vi "write_fifo_resonance_FF_FB.vi"(5 "enable fly-back reversion?":bool, 6 "invert channels":bool[](array[boolean])=[FALSE, FALSE], 7 "fly-back?":bool, 8 "pixel finished?":bool, 10 "maximum bit depth":i8, 11 "integration cluster in":T1) -> (0 "FIFO overflow out":bool, 3 "integration cluster out":T1)   [LabVIEW 2010]
uses:
  integration_cluster.ctl
  <vilib>/rvi/DataTransferAndStorage/Container/XNode/niFpgaContainer.xnode
  <vilib>/rvi/DataTransferAndStorage/Container/Common/niFpgaContainerMethod.ctl
  <vilib>/rvi/DataTransferAndStorage/Container/Common/niFpgaTransferTypeControl.ctl
  <vilib>/rvi/Memory/Memory_Emulation/nirvimemoryEmulationManagerCache_GetValue.vi
  <vilib>/rvi/DataTransferAndStorage/Container/Common/niFpgaContainerGetUniqueNameForEmu.vi
  <vilib>/rvi/Memory/Memory_Emulation/nirvimemoryEmulationManagerCache_InsertValue.vi
  <vilib>/Utility/error.llb/Clear Errors.vi
  <vilib>/rvi/Memory/Memory_Emulation/nirvimemoryEmulationManagerCache_SetValue.vi
  <vilib>/rvi/interface/RandomDataEmulation/nirviRandomDataFPGAFIFO.vi
  <vilib>/rvi/interface/RandomDataEmulation/niFpgaRandomDataHandleErrors.vi
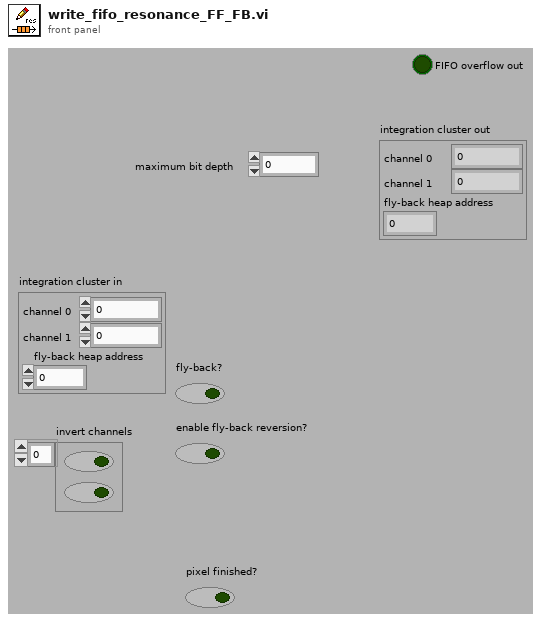
[diagram p1: front panel]
types:
  T1 = typedef "integration_cluster.ctl" = cluster{"channel 0":u32, "channel 1":u32, "fly-back heap address":u32}
  T2 = typedef "niFpgaContainerMethod.ctl" = enum16{"<none>", "write", "read", "clear", "getNumberOfElementsToWrite", "getNumberOfElementsToRead", "enable", "disable", "flushAndDisable", "getStreamState", "readA", "readB", "dramWrite", "dramWriteWithByteEnables", "dramRequestData", "dramRetrieveData"}
  T3 = typedef "niFpgaTransferTypeControl.ctl" = enum16{"Target-Scoped", "Host to Target - DMA", "Target to Host - DMA", "Peer to Peer Reader", "Peer to Peer Writer", "Bidirectional"}
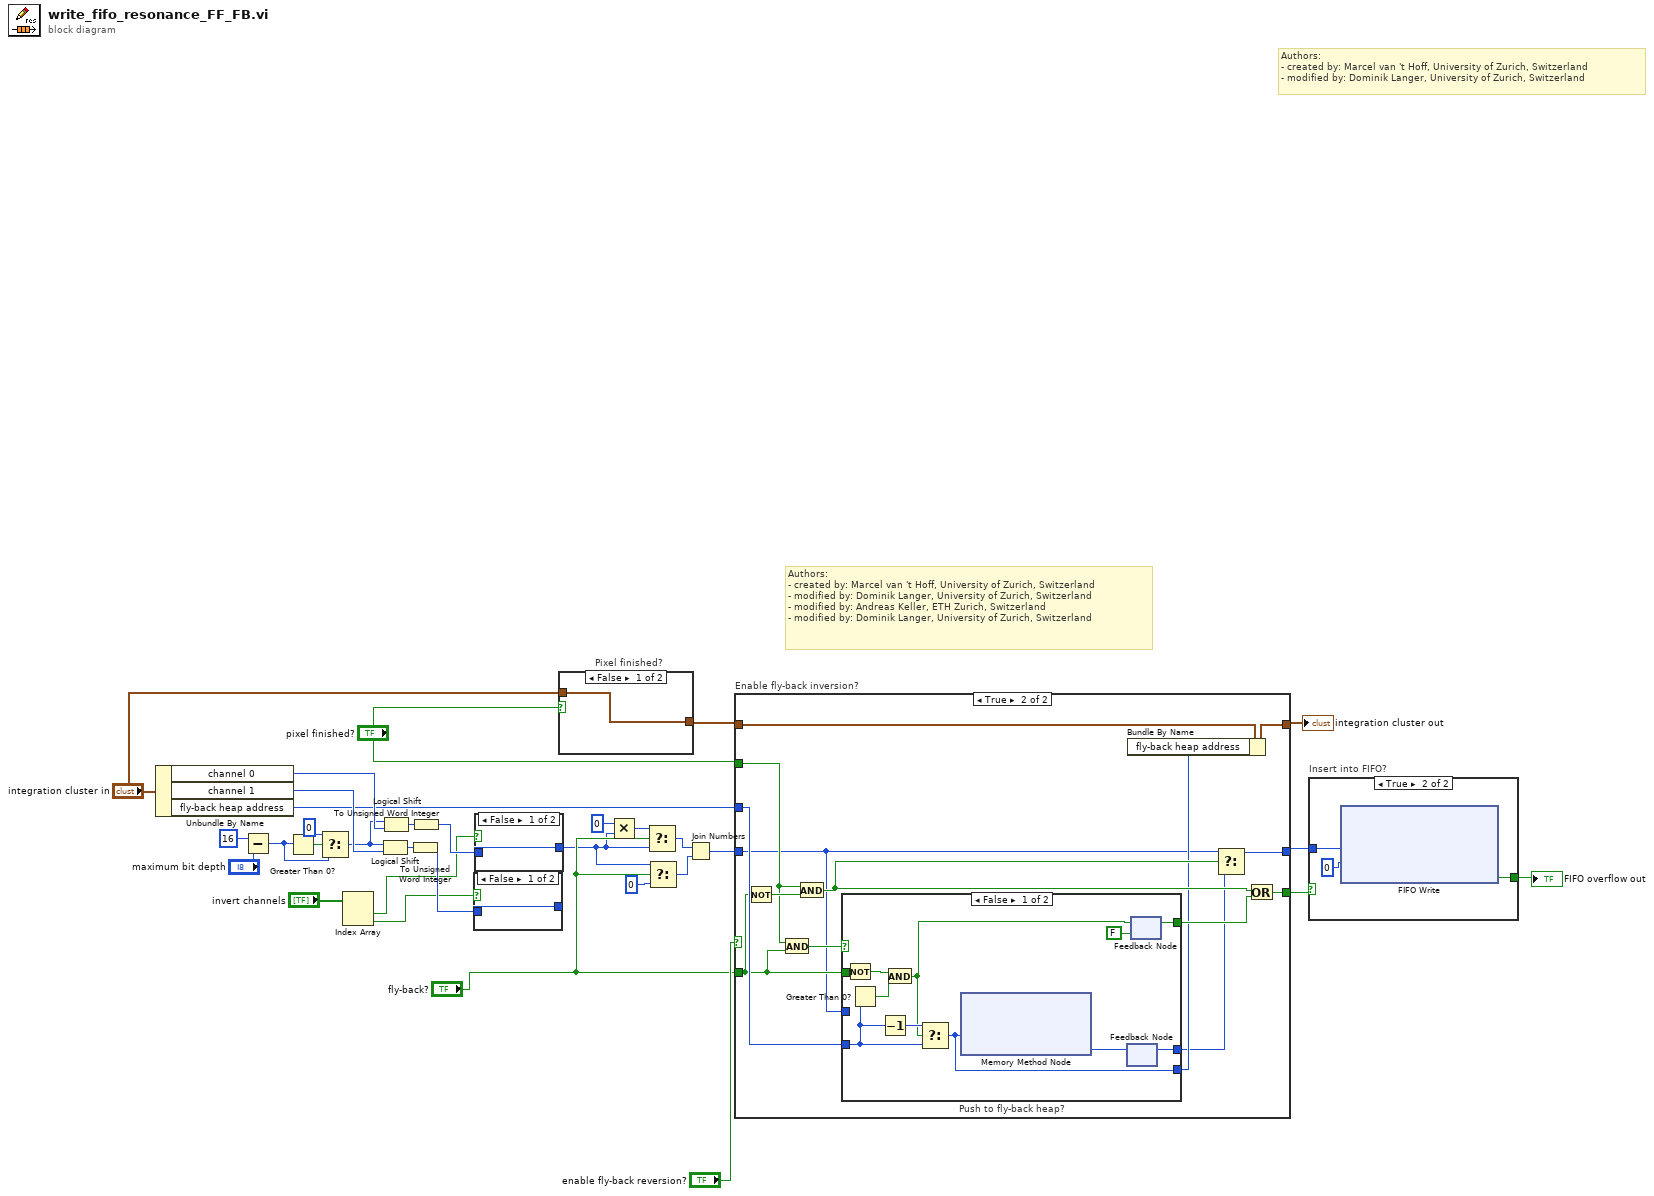
[diagram p0: block diagram]
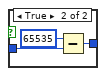
[diagram p2: hidden frame]
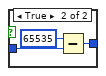
[diagram p3: hidden frame]
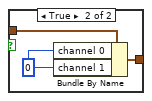
[diagram p4: hidden frame]
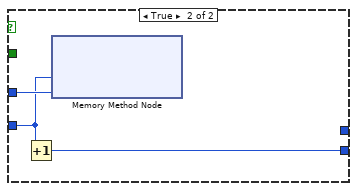
[diagram p6: hidden frame]
diagram:
  # "Authors: \n- created by: Marcel van 't Hoff, University of Zurich, Switzerland\n- modified by: Dominik Langer, University of Zurich, Switzerland\n- modified by: Andreas Keller, ETH Zurich, Switzerland\n- modified by: Dominik Langer, University of Zurich, Switzerland"
  # "Authors: \n- created by: Marcel van 't Hoff, University of Zurich, Switzerland\n- modified by: Dominik Langer, University of Zurich, Switzerland"
  n1 = Unbundle By Name("integration cluster in") -> ("channel 0"=w25:u32, "channel 1"=w26:u32, "fly-back heap address"=w19:u32)
  n2 = Subtract(x=i8 16, y="maximum bit depth") -> (x-y=w28:i8)
  n3 = Greater Than 0?(x=w28) -> (x > 0?=w27:bool)
  n4 = Select(t=i8 0 ("f"), s=w27, f=w28) -> (s? t:f=w24:i8)
  n5 = Index Array(array="invert channels") -> (element #1=w10:bool, element #2=w9:bool)  [unwired: 2 in]
  n6 = Logical Shift(y=w24, x=w26) -> (x << y=w23:u32)
  n7 = Logical Shift(y=w24, x=w25) -> (x << y=w22:u32)
  n8 = To Unsigned Word Integer(number=w23) -> (unsigned 16bit integer=w12:u16)
  n9 = To Unsigned Word Integer(number=w22) -> (unsigned 16bit integer=w13:u16)
  n10 = case shown="False" w9 {
    tunnel: [w33 w35] -> _
    tunnel: w12 -> [w33 w34]
    frame False {
    }
    frame True {
      n11 = Subtract(x=u16 65535, y=w34) -> (x-y=w35:u16)
    }
  }
  n12 = case shown="False" w10 {
    tunnel: [w37 w39] -> w3
    tunnel: w13 -> [w37 w38]
    frame False {
    }
    frame True {
      n13 = Subtract(x=u16 65535, y=w38) -> (x-y=w39:u16)
    }
  }
  n14 = case "Pixel finished?" shown="False" "pixel finished?" {
    tunnel: "integration cluster in" -> [w41 w43]
    tunnel: [w41 w42] -> w16
    frame False {
    }
    frame True {
      w44 = u32 0 ("channel 1")
      n15 = Bundle By Name(cluster=w43, "channel 0"=w44, "channel 1"=w44) -> (w42:T1)
    }
  }
  n16 = Multiply(x=u16 0, y=w3) -> (x*y=w7:u16)
  n17 = Select(t=w7, s="fly-back?", f=w3) -> (s? t:f=w8:u16)
  n18 = Select(t=w3, s="fly-back?", f=u16 0 ("x")) -> (s? t:f=w4:u16)
  n19 = Join Numbers(hi=w8, lo=w4) -> ((hi.lo)=w1:u32)
  n20 = case "Enable fly-back inversion?" shown="True" "enable fly-back reversion?" {
    tunnel: w19 -> [_ w61]
    tunnel: w1 -> [w47 w50]
    tunnel: [w47 w59] -> w21
    tunnel: "pixel finished?" -> [w46 w54]
    tunnel: [w46 w49] -> w18
    tunnel: "fly-back?" -> [_ w56]
    tunnel: w16 -> [w45 w53]
    tunnel: [w45 w51] -> w14
    frame False {
    }
    frame True {
      n21 = Not(x=w56) -> (.not. x?=w60:bool)
      n22 = And(x=w54, y=w56) -> (x .and. y?=w58:bool)
      n23 = And(x=w54, y=w60) -> (x .and. y?=w57:bool)
      n24 = case "Push to fly-back heap?" shown="False" w58 {
        tunnel: w50 -> [_ w201]
        tunnel: [w64 w200] -> w52
        tunnel: w61 -> [w66 w199]
        tunnel: w56 -> [w71 _]
        tunnel: [w68 _] -> w48
        tunnel: [w70 _] -> w55
        frame False {
          n25 = Not(x=w71) -> (.not. x?=w63:bool)
          n26 = Greater Than 0?(x=w66) -> (x > 0?=w72:bool)
          n27 = Decrement(x=w66) -> (x-1=w65:u32)
          n28 = And(x=w63, y=w72) -> (x .and. y?=w62:bool)
          n29 = Select(t=w65, s=w62, f=w66) -> (s? t:f=w64:u32)
          n30 = xnode ("Memory Method Node")("Address"=w64) -> ("Data"=w67:u32)  [unwired: 1 in, 1 out]
          n31 = feedback #1() -> (w68:u32)  [unwired: 1 in]
          n32 = feedback-in #1(w67) -> ()
          n33 = feedback #2(FALSE) -> (w70:bool)
          n34 = feedback-in #2(w62) -> ()
        }
        frame True {
          n35 = Increment(x=w199) -> (x+1=w200:u32)
          n36 = xnode ("Memory Method Node")("Address"=w199, "Data"=w201) -> ()  [unwired: 1 in, 1 out]
        }
      }
      n37 = Bundle By Name(cluster=w53, "fly-back heap address"=w52) -> (w51:T1)
      n38 = Select(t=w50, s=w57, f=w48) -> (s? t:f=w59:u32)
      n39 = Or(x=w57, y=w55) -> (x .or. y?=w49:bool)
    }
  }
  "integration cluster out" <- w14
  n40 = case "Insert into FIFO?" shown="True" w18 {
    tunnel: [_ w329] -> w31
    tunnel: w21 -> [_ w327]
    frame False {
    }
    frame True {
      n41 = xnode ("FIFO Write")("Element"=w327, "Timeout"=0) -> ("Timed Out?"=w329:bool)  [unwired: 1 in, 1 out]
    }
  }
  "FIFO overflow out" <- w31
